vi "Parser_0xE6_(SubVI).vi"(11 "String in":string) -> (1 "length":i32, 2 "Array":sgl[](array[numeric]))   [LabVIEW 2017, in "LV_Unicorn.lvlib"]
uses:
  LV_Unicorn.lvlib
panel:
  out "Array 2":string[](array[string])
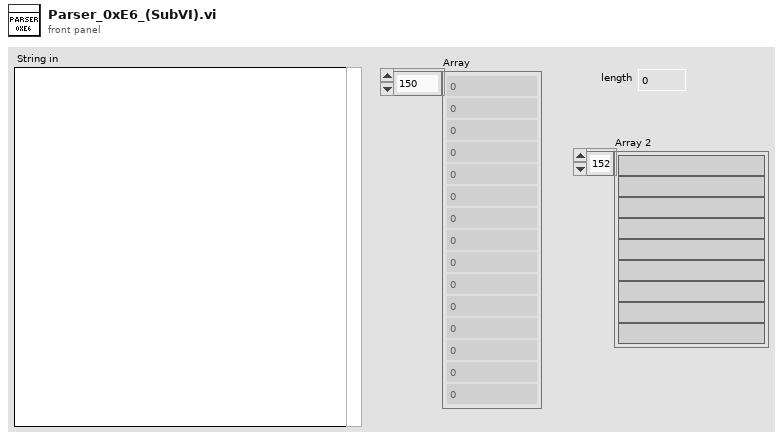
[diagram p1: front panel]
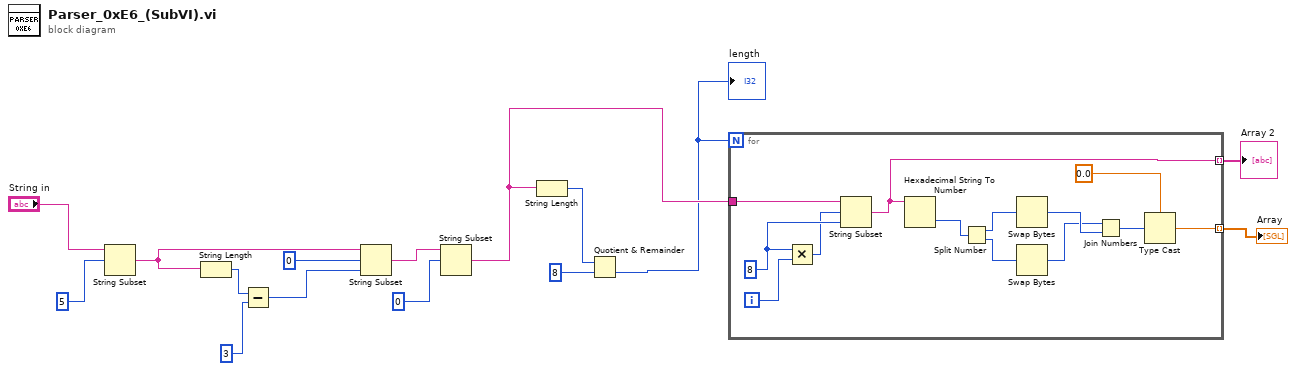
[diagram p0: block diagram]
diagram:
  n1 = String Subset(string="String in", offset (0)=5) -> (substring=w3:string)  [unwired: 1 in]
  n2 = String Length(string=w3) -> (length=w12:i32)
  n3 = Subtract(x=w12, y=3) -> (x-y=w4:i32)
  n4 = String Subset(string=w3, offset (0)=0, length (rest)=w4) -> (substring=w5:string)
  n5 = String Subset(string=w5, offset (0)=0) -> (substring=w9:string)  [unwired: 1 in]
  n6 = String Length(string=w9) -> (length=w8:i32)
  n7 = Quotient & Remainder(x=w8, y=8) -> (floor(x/y)=w1:i32)  [unwired: 1 out]
  "length" <- w1
  n8 = for {
    N: w1 -> [_]
    tunnel: w9 -> [w28]
    tunnel: [w17] -> w6 mode=indexing
    tunnel: [w16] -> w2 mode=indexing
    i -> [w20]
    w19 = 8 ("length (rest)")
    n9 = Multiply(x=w19, y=w20) -> (x*y=w18:i32)
    n10 = String Subset(string=w28, offset (0)=w18, length (rest)=w19) -> (substring=w16:string)
    n11 = Hexadecimal String To Number(string=w16) -> (number=w26:u32)  [unwired: 2 in, 1 out]
    n12 = Split Number(x=w26) -> (hi(x)=w25:u16, lo(x)=w24:u16)
    n13 = Swap Bytes(anything=w25) -> (byte swapped=w23:u16)
    n14 = Swap Bytes(anything=w24) -> (byte swapped=w22:u16)
    n15 = Join Numbers(hi=w22, lo=w23) -> ((hi.lo)=w21:u32)
    n16 = Type Cast(type=sgl 0.0, x=w21) -> (*(type *) &x=w17:sgl)
  }
  "Array" <- w6
  "Array 2" <- w2
